vi "Test Get Inherited Test Name.vi"(8 "error in (no error)":errorcluster, 11 "Test Case In":refnum<class "Inheritance Test.lvclass">) -> (0 "error out":errorcluster, 3 "Test Case Out":refnum<class "Inheritance Test.lvclass">)   [LabVIEW 2020, in "Inheritance Test.lvclass"]
uses:
  Inheritance Test.lvclass
  C:/Program Files (x86)/National Instruments/LabVIEW 2020/vi.lib/Astemes/LUnit/Test Case.lvclass
  Test Doubles/Test Case Test Double/Test Case Test Double Child.lvclass
  Test Doubles/Test Case Test Double Parent/Test Case Test Double Parent.lvclass
  <vilib>/Astemes/LUnit/Test Case.lvclass/Test Case.ctl
  e8c5eeff-a694-4c0d-b261-74e2e6f5327d.vi
  <vilib>/Astemes/LUnit/Append Pass Result.vi
  <vilib>/Astemes/LUnit/Append Fail Result.vi
  <vilib>/Astemes/LUnit/Describe Comparison.vi
  <vilib>/Astemes/LUnit/Compare Variants.vi
  <vilib>/Astemes/LUnit/Run In UI.vi
  <vilib>/Utility/error.llb/Clear Errors.vi
  <vilib>/Utility/LVClass/Get LV Class Name.vi
  <vilib>/Astemes/LUnit/Describe Variant.vi
  <vilib>/Astemes/LUnit/Test Case.lvclass
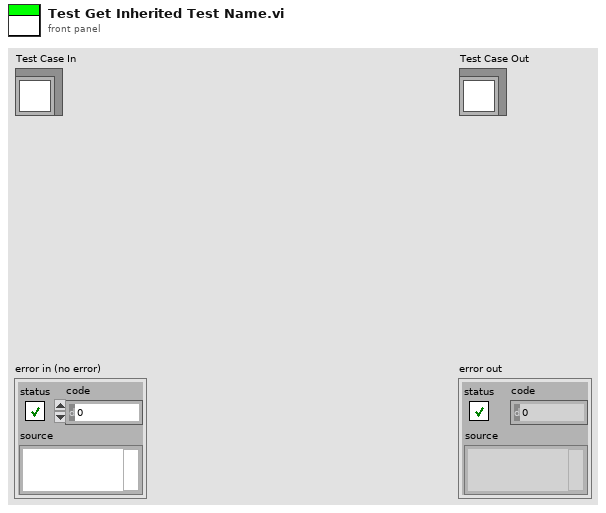
[diagram p1: front panel]
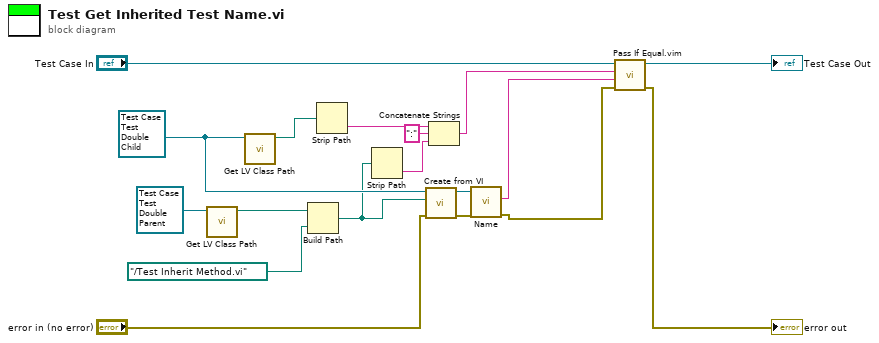
[diagram p0: block diagram]
diagram:
  w3 = refnum<class "Test Case Test Double Child.lvclass"> refnum ("Test Case Test Double Child.lvclass")
  n1 = call <vilib>:"Get LV Class Path.vi"("object"=refnum<class "Test Case Test Double Parent.lvclass"> refnum ("Test Case Test Double Parent.lvclass")) -> ("class path"=w9:path)  [unwired: 9 in, 1 out]
  n2 = call <vilib>:"Get LV Class Path.vi"("object"=w3) -> ("class path"=w8:path)  [unwired: 9 in, 1 out]
  n3 = Build Path(base path=w9, name or relative path=path "../Test Inherit Method.vi" ("Relative Path from 1 to 2")) -> (appended path=w2:path)
  n4 = Strip Path(path=w8) -> (name=w7:string)  [unwired: 1 out]
  n5 = Strip Path(path=w2) -> (name=w5:string)  [unwired: 1 out]
  n6 = call <vilib>:"Create from VI.vi"("error in (no error)"="error in (no error)", "Test Method VI Path"=w2, "LUnit Test Case Class"=w3) -> ("error out"=w13:errorcluster, "LUnit Test Case Out"=w14:refnum<class "Test Case Test Double Child.lvclass">)  [unwired: 7 in]
  n7 = Concatenate Strings(w7, ":" ("string"), w5) -> (w4:string)
  n8 = call-dynamic "Name.vi"("error in (no error)"=w13, "LUnit Test Case in"=w14) -> ("error out"=w11:errorcluster, "Name"=w12:string)  [unwired: 7 in, 1 out]
  n9 = call "Pass If Equal.vim"("error in (no error)"=w11, "Actual"=w12, "Expected"=w4, "LUnit Test Case In"="Test Case In") -> ("error out"=→"error out":errorcluster, "LUnit Test Case Out"=→"Test Case Out":refnum<class "Inheritance Test.lvclass">)  [unwired: 6 in]
